vi "Test New Sweep.vi"() -> ()   [LabVIEW 2016, in "Lockin.DAQ.lvclass"]
uses:
  Lockin.DAQ.lvclass
  Typedefs/Sweep Pattern--Enum.ctl
  <vilib>/Analysis/1siggen.llb/Ramp Pattern by Samples.vi
  <vilib>/Analysis/NI_AALBase.lvlib
panel:
  in  "Sweep Lockin Time (s)":dbl=10.0 format="%#_13g"
  in  "Sweep Type":T1[](array[typedef])
  in  "milliseconds to wait":u32
  out "XY Graph 2":cluster{"Ramp Pattern":dbl[], dbl[]}[](graph)
  out "XY Graph":T2(graph)
  out "Numeric 2":i32
  out "Numeric 1":i32
  out "Numeric 3":i32
  in  "DC":dbl[](array[numeric])
  in  "Sweep Channel":i32[](array[numeric])
  in  "Sweep End":dbl[](array[numeric])
  in  "Sweep Start":dbl[](array[numeric])
  out "End (V)":dbl[](array[numeric])
  out "Start (V)":dbl[](array[numeric])
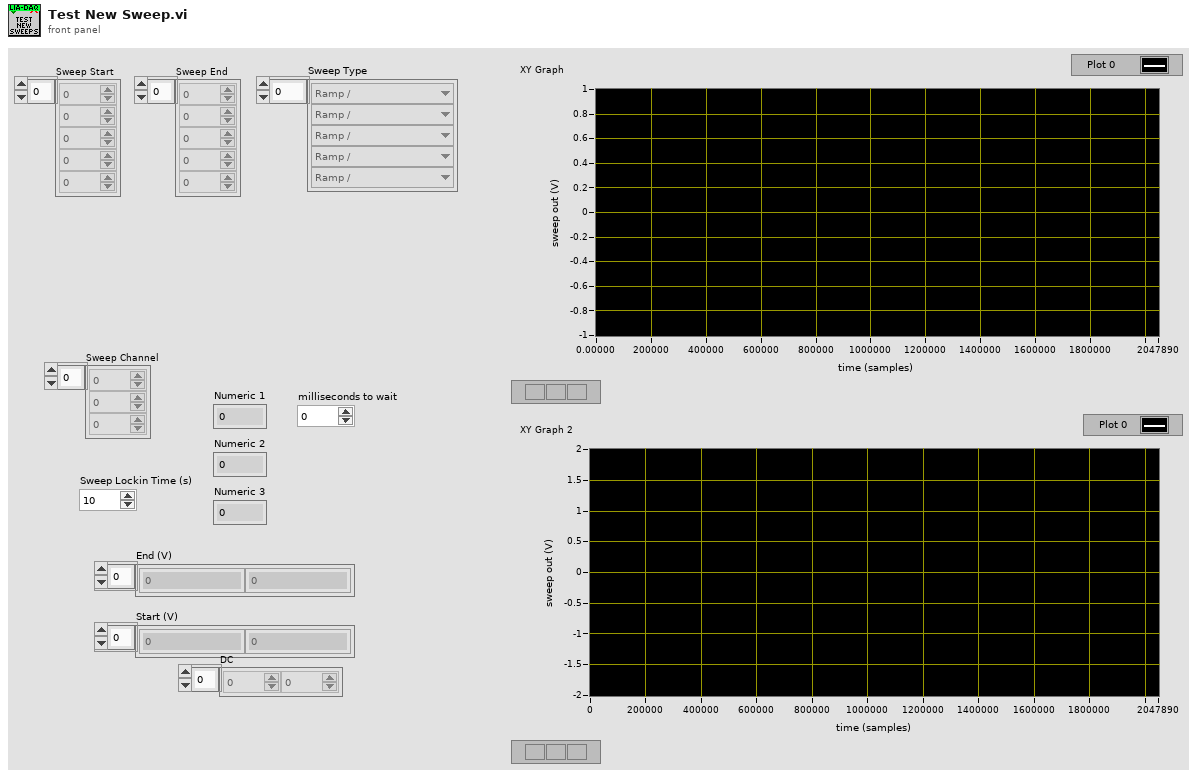
[diagram p1: front panel]
types:
  T1 = typedef "Lockin.DAQ.lvclass/Sweep Pattern--Enum.ctl" = enum16{"Ramp /", "Ramp /\\", "Smooth Ramp _/", "Smooth Ramp _/\\_", "Frequency"}
  T2 = cluster{"Ramp Pattern":dbl[], "Ramp Pattern":dbl[]}[]
  T3 = cluster{"Ramp Pattern":dbl[], "output waveform":waveform(dbl)}
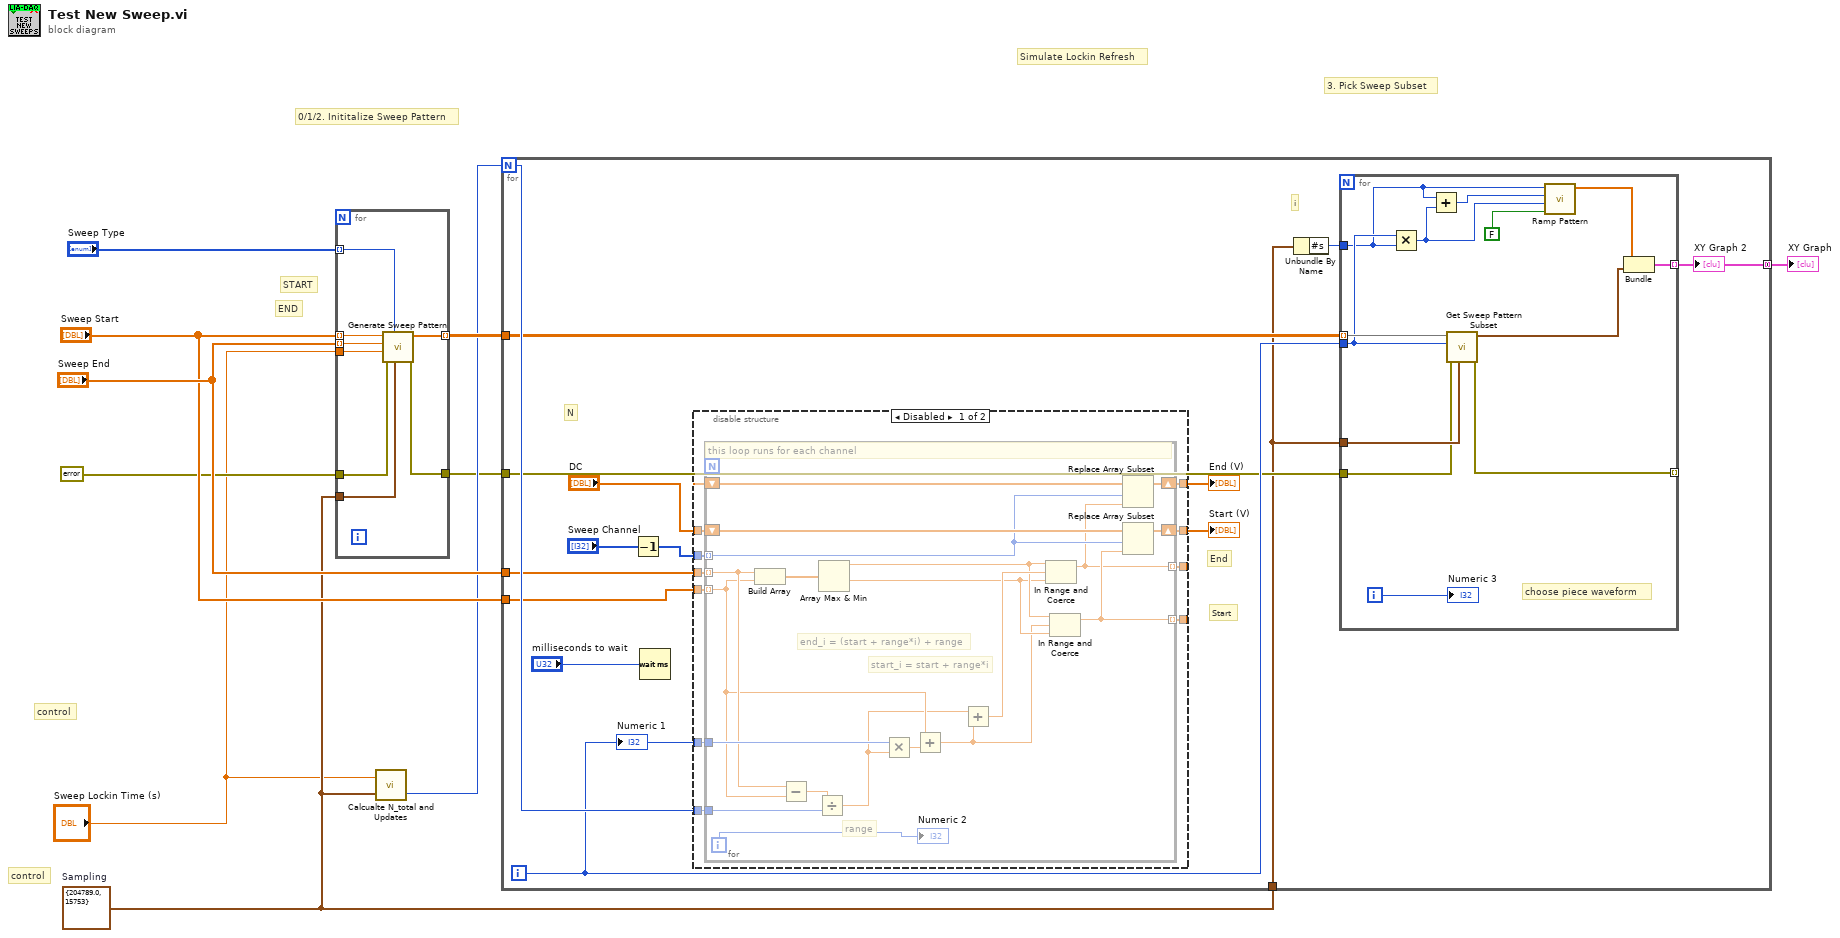
[diagram p0: block diagram]
diagram:
  w4 = cluster{"Fs":dbl, "#s":i32} {"Fs"=204789.0, "#s"=15753}  # Sampling
  # "3. Pick Sweep Subset"
  # "Simulate Lockin Refresh"
  # "0/1/2. Inititalize Sweep Pattern"
  # "END"
  # "START"
  # "control"
  # "control"
  n1 = for {
    tunnel: "Sweep Start" -> [w17] mode=indexing
    tunnel: "Sweep End" -> [w18] mode=indexing
    tunnel: [w16] -> w7 mode=indexing
    tunnel: "Sweep Type" -> [w11] mode=indexing
    tunnel: [w12] -> w1
    tunnel: errorcluster {"status"=FALSE, "code"=0, "source"=""} ("error in (no error)") -> [w13]
    tunnel: w4 -> [w14]
    tunnel: "Sweep Lockin Time (s)" -> [w15]
    n2 = call "Generate Sweep Pattern.vi"("Sampling"=w14, "Sweep Pattern"=w11, "error in (no error)"=w13, "Sweep Lockin Time (s)"=w15, "Sweep End"=w18, "Sweep Start"=w17) -> ("error out"=w12:errorcluster, "Sweep Pattern"=w16:dbl[])  [unwired: 4 in]
  }
  n3 = call "Calcualte N_total and Updates.vi"("Sampling"=w4, "Sweep Time (s)"="Sweep Lockin Time (s)") -> ("Updates"=w3:i32)  [unwired: 1 out]
  n4 = for {
    N: w3 -> [w28]
    tunnel: w4 -> [w19]
    tunnel: "Sweep Start" -> [w26]
    tunnel: "Sweep End" -> [w25]
    tunnel: w7 -> [w23]
    tunnel: [w21] -> w8 mode=concatenating
    tunnel: w1 -> [w20]
    i -> [w27]
    # "i"
    # "Start"
    # "End"
    # "N"
    n5 = Decrement(x="Sweep Channel") -> (x-1=w33:i32[])
    n6 = Wait (ms)(milliseconds to wait="milliseconds to wait") -> ()  [unwired: 1 out]
    n7 = disable-structure shown="Disabled" {
      disable-tunnel: w33 -> [w43 _]
      disable-tunnel: "DC" -> [w42 _]
      disable-tunnel: [w41 _] -> w31
      disable-tunnel: [w40 _] -> w30
      disable-tunnel: [w39 _] -> _
      disable-tunnel: [w38 _] -> _
      disable-tunnel: w28 -> [w37 _]
      disable-tunnel: w27 -> [w36 _]
      disable-tunnel: w26 -> [w35 _]
      disable-tunnel: w25 -> [w34 _]
      frame Disabled {
        n8 = for {
          shift-right: [w62] -> w41
          shift-left: w42 -> [w63]
          shift-right: [w60] -> w40
          shift-left: w42 -> [w61]
          tunnel: w35 -> [w46] mode=indexing
          tunnel: w34 -> [w54] mode=indexing
          tunnel: w43 -> [w55] mode=indexing
          tunnel: w36 -> [w57]
          tunnel: w37 -> [w59]
          tunnel: [w50] -> w38 mode=indexing
          tunnel: [w49] -> w39 mode=indexing
          i -> [w45]
          # "end_i = (start + range*i) + range"
          # "start_i = start + range*i"
          # "range"
          # "this loop runs for each channel"
          n9 = Build Array(w54, w46) -> (w53:dbl[])
          n10 = Subtract(x=w54, y=w46) -> (x-y=w48:dbl)
          n11 = Divide(x=w48, y=w59) -> (x/y=w44:dbl)
          n12 = Array Max & Min(array=w53) -> (max value=w52:dbl, min value=w51:dbl)  [unwired: 2 out]
          n13 = Multiply(x=w57, y=w44) -> (x*y=w58:dbl)
          n14 = Add(x=w46, y=w58) -> (x+y=w47:dbl)
          n15 = Add(x=w44, y=w47) -> (x+y=w56:dbl)
          n16 = In Range and Coerce(upper limit=w52, x=w56, lower limit=w51) -> (coerced(x)=w49:dbl)  [unwired: 1 out]
          n17 = In Range and Coerce(upper limit=w52, x=w47, lower limit=w51) -> (coerced(x)=w50:dbl)  [unwired: 1 out]
          n18 = Replace Array Subset(array=w63, new element=w49, index=w55) -> (w62:dbl[])
          n19 = Replace Array Subset(array=w61, new element=w50, index=w55) -> (w60:dbl[])
          "Numeric 2" <- w45
        }
      }
      frame Enabled {
      }
    }
    "Start (V)" <- w30
    "End (V)" <- w31
    n20 = Unbundle By Name(w19) -> ("#s"=w29:i32)
    n21 = for {
      tunnel: w29 -> [w67]
      tunnel: [w74] -> w21 mode=indexing
      tunnel: w27 -> [w68]
      tunnel: w23 -> [w73] mode=indexing
      tunnel: w20 -> [w65]
      tunnel: [w64] -> _ mode=indexing
      tunnel: w19 -> [w66]
      i -> [w76]
      # "choose piece waveform"
      n22 = Multiply(x=w68, y=w67) -> (x*y=w69:i32)
      n23 = Add(x=w67, y=w69) -> (x+y=w70:i32)
      n24 = call "Get Sweep Pattern Subset.vi"("Sampling"=w66, "error in (no error)"=w65, "index"=w68, "Sweep Pattern"=w73) -> ("error out"=w64:errorcluster, "output waveform"=w72:waveform(dbl))  [unwired: 5 in, 1 out]
      n25 = call-poly <vilib>:"Ramp Pattern.vi"("exclude end?"=FALSE, "start"=w69, "end"=w70, "samples"=w67) -> ("Ramp Pattern"=w75:dbl[])  [unwired: 6 in, 1 out]
      n26 = Bundle("Ramp Pattern"=w75, "output waveform"=w72) -> (w74:T3)  [unwired: 1 in]
      "Numeric 3" <- w76
    }
    "XY Graph 2" <- w21
    "Numeric 1" <- w27
  }
  "XY Graph" <- w8
